vi "配置变量_temp.vi"() -> ()   [LabVIEW 2014]
panel:
  in  "主界面配置":T1={"侧边栏数据"=[], "界面刷间隔率"=1000.0}
  in  "compactRIO配置":T2
  in  "应用信息":T3(array[cluster])
  in  "show配置":T4
  in  "测试模块8":T5(array[cluster])
  in  "测试模块7":T5(array[cluster])
  in  "测试模块6":T5(array[cluster])
  in  "测试模块5":T5(array[cluster])
  in  "测试模块4":T5(array[cluster])
  in  "测试模块3":T5(array[cluster])
  in  "测试模块2":T5(array[cluster])
  in  "测试模块1":T5(array[cluster])
  in  "cRIO模块":T5(array[cluster])
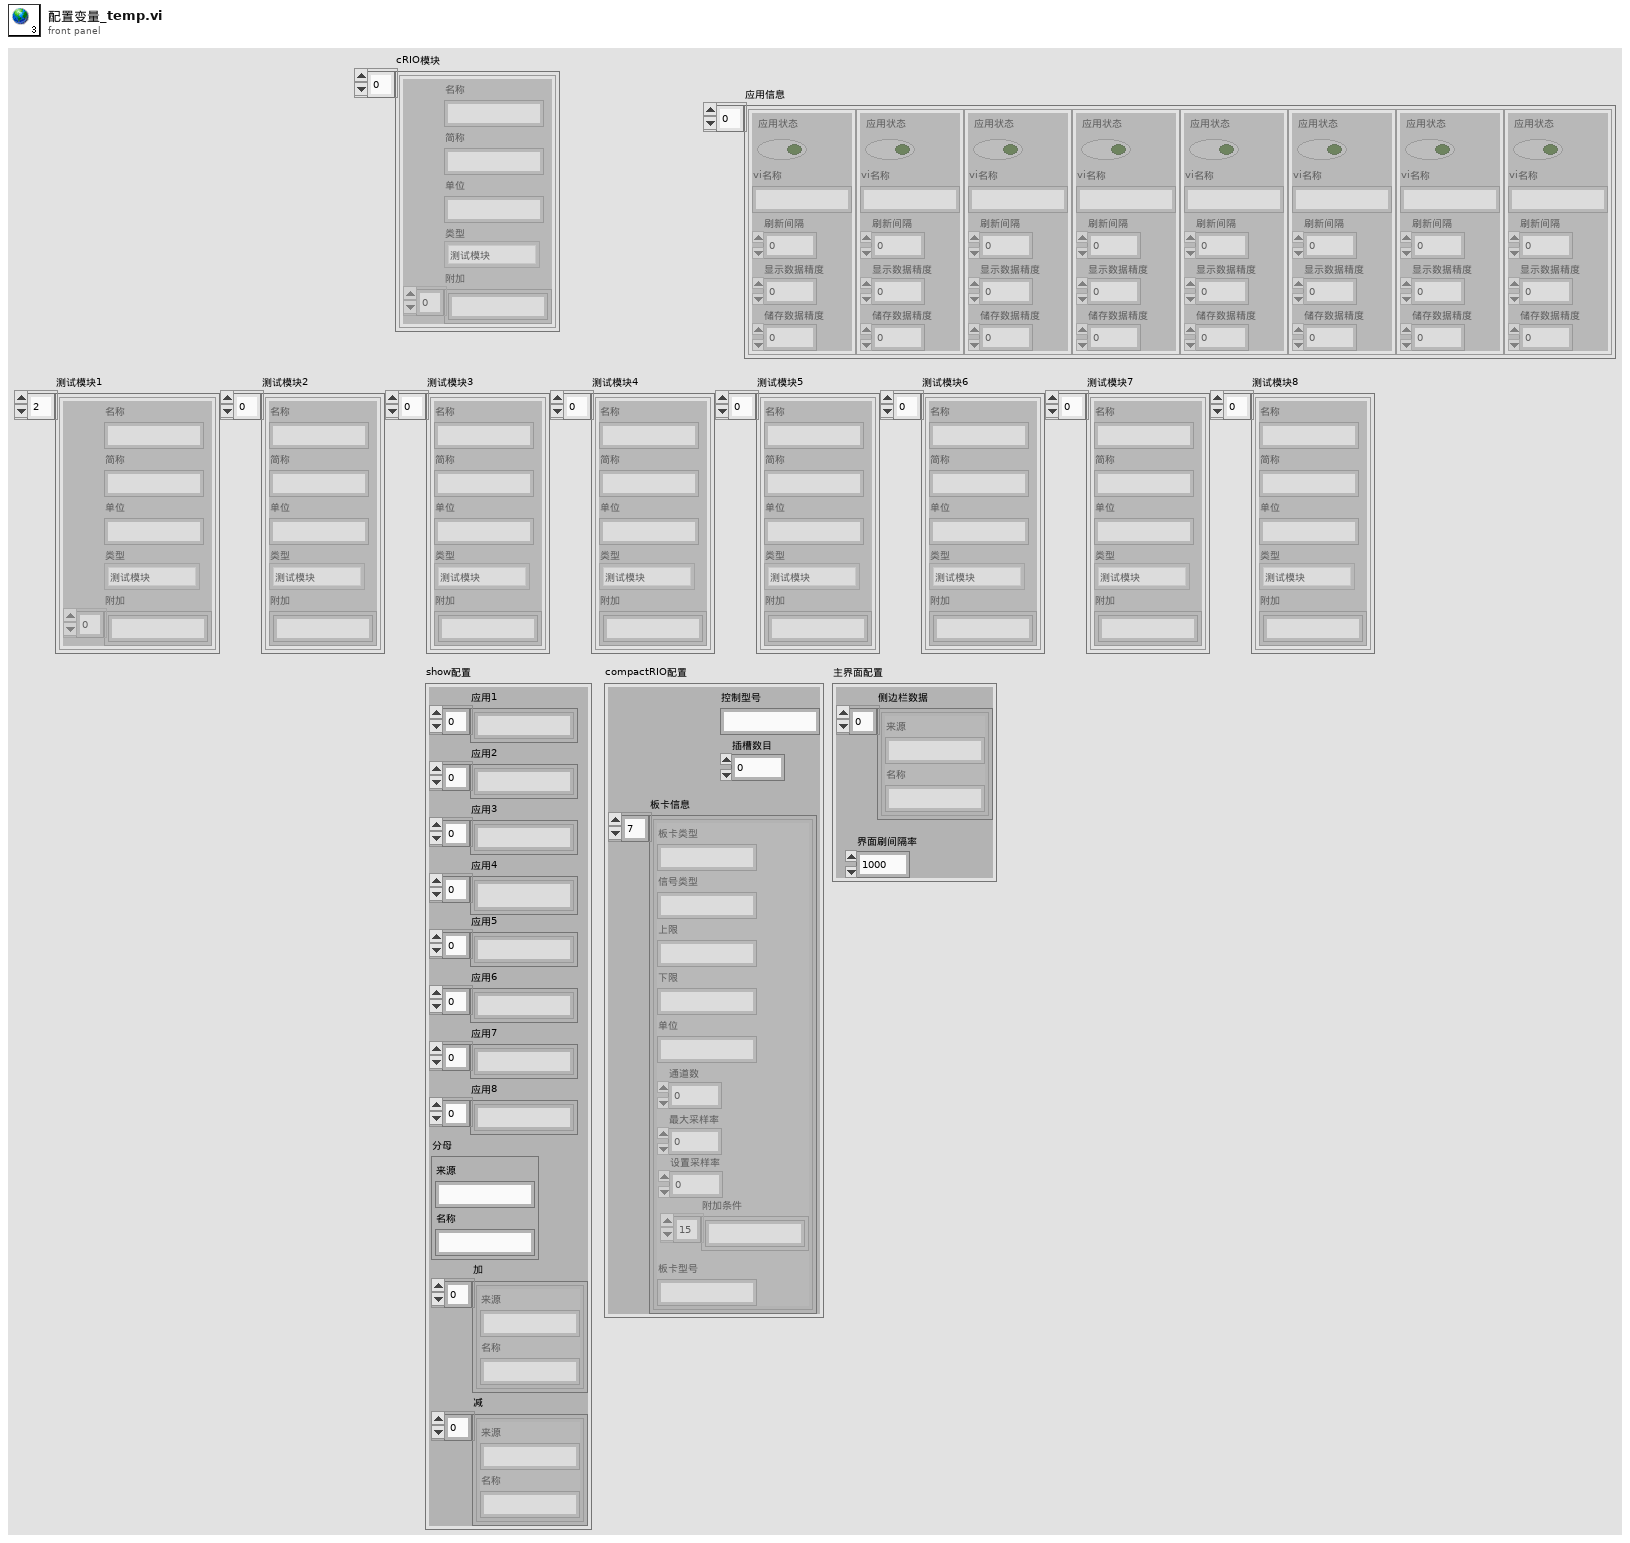
[diagram p1: front panel]
types:
  T1 = cluster{"侧边栏数据":cluster{"来源":string, "名称":string}[], "界面刷间隔率":dbl}
  T2 = cluster{"控制型号":string, "插槽数目":u32, "板卡信息":cluster{"板卡类型":string, "信号类型":string, "上限":string, "下限":string, "单位":string, "通道数":u32, "最大采样率":u32, "设置采样率":u32, "附加条件":string[], "板卡型号":string}[]}
  T3 = cluster{"应用状态":bool, "vi名称":string, "刷新间隔":u32, "显示数据精度":u32, "储存数据精度":u32}[]
  T4 = cluster{"应用1":string[], "应用2":string[], "应用3":string[], "应用4":string[], "应用5":string[], "应用6":string[], "应用7":string[], "应用8":string[], "分母":cluster{"来源":string, "名称":string}, "加":cluster{"来源":string, "名称":string}[], "减":cluster{"来源":string, "名称":string}[]}
  T5 = cluster{"名称":string, "简称":string, "单位":string, "附加":string[], "类型":enum16{"测试模块", "FPGA", "cRIO", "其他设备", "总体展示"}}[]
diagram:
